vi "DOCK_add_batch_ID_pair_to_batch_ID_buffer.vi"(6 "SQL_result":variant, 8 "error_in":errorcluster, 10 "BATCH_CODE":string, 11 "SQL_pinion_ID_buffer_all_info_in":T1) -> (0 "error_out":errorcluster, 1 "BATCH_ID_out":string, 2 "Batch exists?":bool, 3 "SQL_pinion_ID_buffer_all_info_out":T1)   [LabVIEW 2019]
uses:
  DOCK_batch_ID_buffer_all_info.ctl
  _misc/AULocalize/SubVIs/Get Localized Phrase Compact Interface 0D.vi
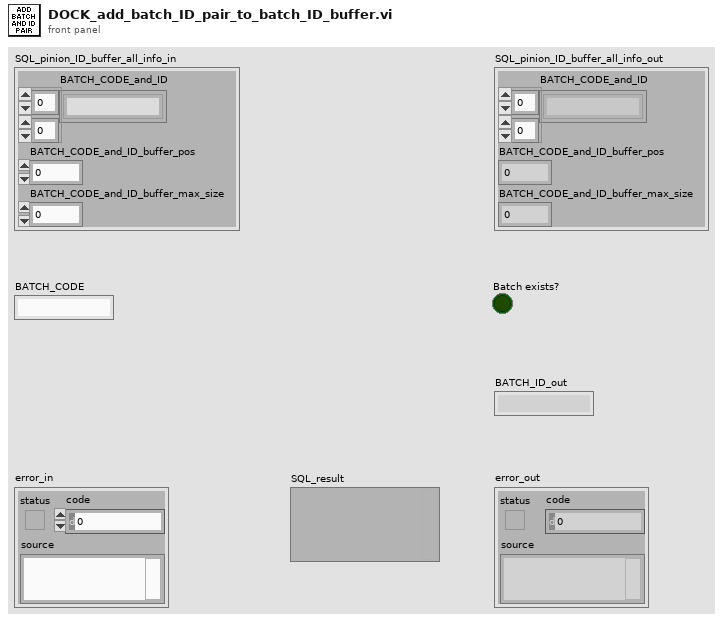
[diagram p1: front panel]
types:
  T1 = typedef "DOCK_batch_ID_buffer_all_info.ctl" = cluster{"BATCH_CODE_and_ID":string[][], "BATCH_CODE_and_ID_buffer_pos":i32, "BATCH_CODE_and_ID_buffer_max_size":i32}
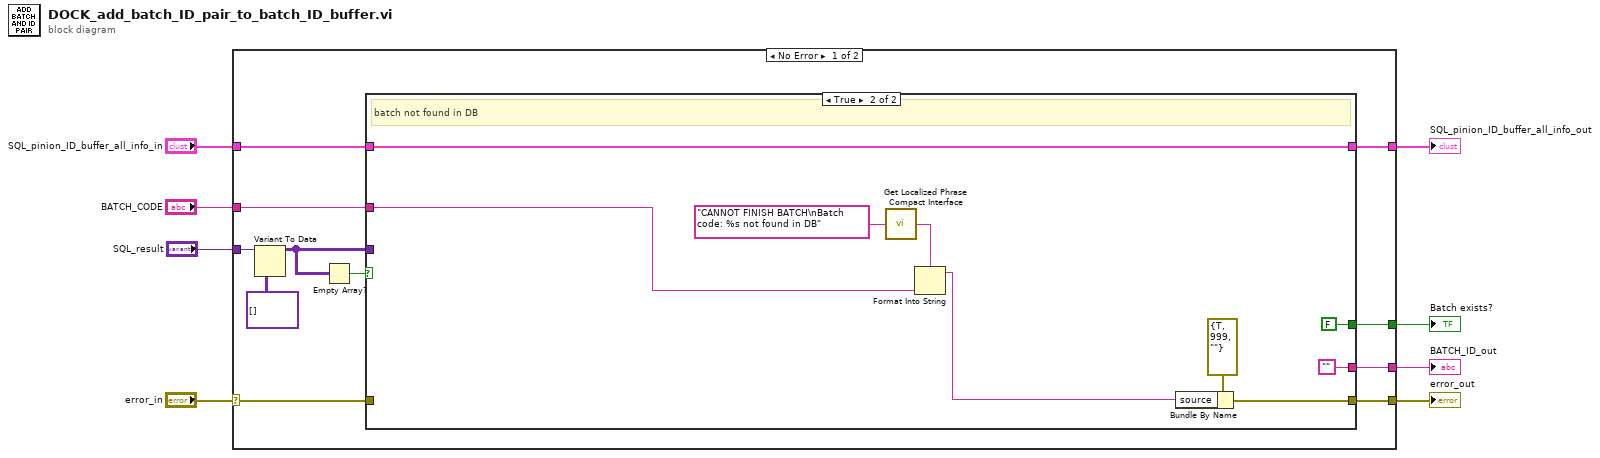
[diagram p0: block diagram]
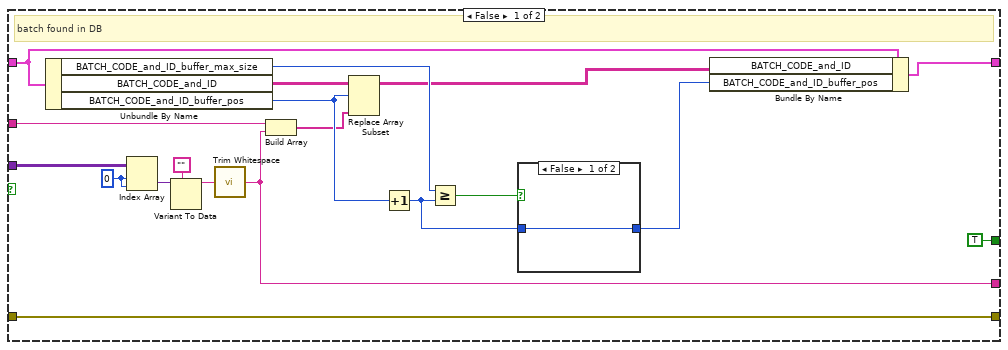
[diagram p2: hidden frame]
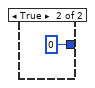
[diagram p3: hidden frame]
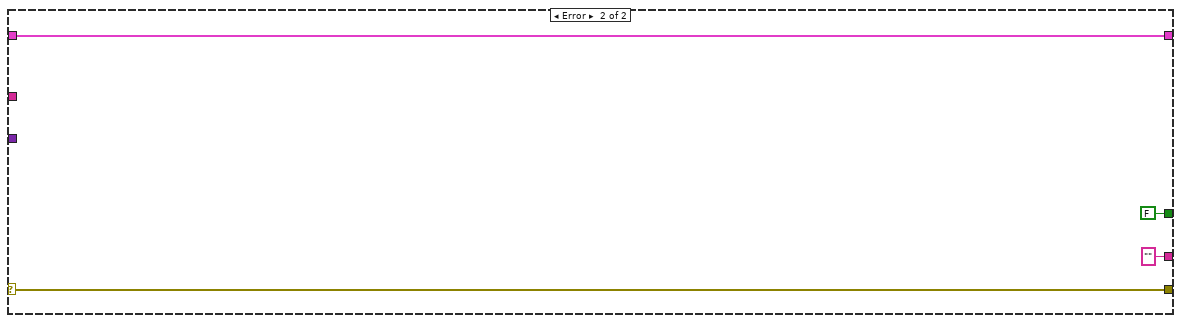
[diagram p4: hidden frame]
diagram:
  n1 = case shown="No Error" "error_in" {
    selector: "error_in" -> [w15 w53]
    tunnel: [w19 w52] -> w8
    tunnel: "SQL_pinion_ID_buffer_all_info_in" -> [w18 w52]
    tunnel: "BATCH_CODE" -> [w17 _]
    tunnel: [w14 w53] -> w4
    tunnel: "SQL_result" -> [w11 _]
    tunnel: [w16 "" ("trimmed string")] -> w3
    tunnel: [w13 FALSE] -> w2
    frame No Error {
      n2 = Variant To Data(type=variant[][] [] ("recordset_in"), Variant=w11) -> (data=w10:variant[][])  [unwired: 1 in, 1 out]
      n3 = Empty Array?(array=w10) -> (empty?=w12:bool)
      n4 = case shown="True" w12 {
        tunnel: [w32 w49] -> w19
        tunnel: w18 -> [w31 w49]
        tunnel: w17 -> [w29 w44]
        tunnel: w10 -> [w23 _]
        tunnel: [w22 ""] -> w16
        tunnel: w15 -> [w21 _]
        tunnel: [w21 w42] -> w14
        tunnel: [TRUE FALSE] -> w13
        frame False {
          w24 = 0 ("index")
          # "batch found in DB"
          n5 = Unbundle By Name(w31) -> ("BATCH_CODE_and_ID_buffer_max_size"=w36:i32, "BATCH_CODE_and_ID"=w28:string[][], "BATCH_CODE_and_ID_buffer_pos"=w34:i32)
          n6 = Index Array(array=w23, index (row)=w24, index (col)=w24) -> (element=w25:variant)
          n7 = Variant To Data(type="", Variant=w25) -> (data=w26:string)  [unwired: 1 in, 1 out]
          n8 = call <vilib>:"Trim Whitespace.vi"("string"=w26) -> ("trimmed string"=w22:string)  [unwired: 1 in]
          n9 = Build Array(w29, w22) -> (w30:string[])
          n10 = Replace Array Subset(array=w28, new element=w30, index (row)=w34) -> (w33:string[][])  [unwired: 1 in]
          n11 = Increment(x=w34) -> (x+1=w37:i32)
          n12 = Greater Or Equal?(x=w36, y=w37) -> (x >= y?=w35:bool)
          n13 = case shown="False" w35 {
            tunnel: w37 -> [w39 _]
            tunnel: [w39 0] -> w38
            frame False {
            }
            frame True {
            }
          }
          n14 = Bundle By Name(cluster=w31, "BATCH_CODE_and_ID"=w33, "BATCH_CODE_and_ID_buffer_pos"=w38) -> (w32:T1)
        }
        frame True {
          # "batch not found in DB"
          n15 = call-poly "Get Localized Phrase Compact Interface.vi"("Key"="CANNOT FINISH BATCH\nBatch code: %s not found in DB") -> ("Translated Phrase"=w41:string)
          n16 = Format Into String(format string=w41, w44) -> (resulting string=w43:string)  [unwired: 2 in, 1 out]
          n17 = Bundle By Name(cluster=errorcluster {"status"=TRUE, "code"=999, "source"=""} ("error IO"), "source"=w43) -> (w42:errorcluster)
        }
      }
    }
    frame Error {
    }
  }
  "SQL_pinion_ID_buffer_all_info_out" <- w8
  "error_out" <- w4
  "BATCH_ID_out" <- w3
  "Batch exists?" <- w2
